vi "specCluster_FGV2.vi"(7 "command":T1, 8 "error in (no error)":errorcluster, 10 "index":i32, 11 "spec cluster":cluster{"dp [MeV/C]":dbl[], dbl[]}) -> (0 "error out":errorcluster, 3 "specArray":T2[](array[typedef]))   [LabVIEW 2011]
uses:
  specCluster_Typdef.ctl
  specClustercommandTypdef.ctl
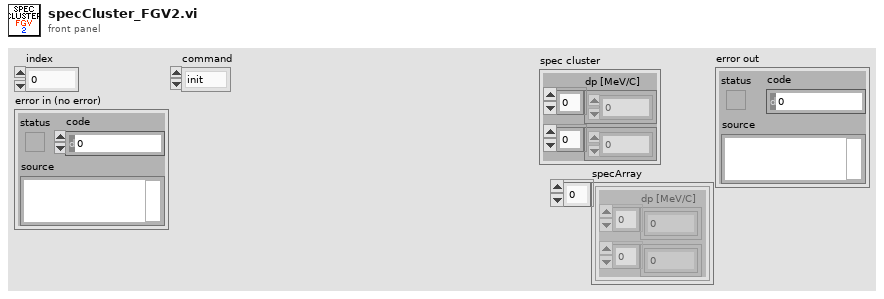
[diagram p1: front panel]
types:
  T1 = typedef "specClustercommandTypdef.ctl" = enum16{"init", "addCluster", "read"}
  T2 = typedef "specCluster_Typdef.ctl" = cluster{"dp [MeV/C]":dbl[], dbl[]}
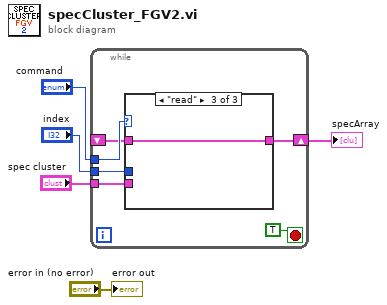
[diagram p0: block diagram]
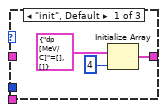
[diagram p2: hidden frame]
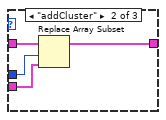
[diagram p3: hidden frame]
diagram:
  n1 = while {
    tunnel: "command" -> [w10]
    shift-right: [w9] -> w2
    shift-left: _ -> [w8]
    tunnel: "spec cluster" -> [w6]
    tunnel: "index" -> [w7]
    stop <- TRUE stop-if-true
    n2 = case shown="\"read\"" w10 {
      tunnel: [w12 w15 w19] -> w9
      tunnel: w8 -> [_ w18 w19]
      tunnel: w7 -> [_ w17 _]
      tunnel: w6 -> [_ w16 _]
      frame "init", Default {
        n3 = Initialize Array(T2 {"dp [MeV/C]"=[], []} ("spec cluster 2"), 4 ("dimension size")) -> (w12:T2[])
      }
      frame "addCluster" {
        n4 = Replace Array Subset(array=w18, new element=w16, index=w17) -> (w15:T2[])
      }
      frame "read" {
      }
    }
  }
  "specArray" <- w2
  "error out" <- "error in (no error)"
